vi "BASE-Julian Code.vi"() -> (0 "Long Date":string, 1 "Short Date":string, 2 "Shift":string, 3 "Julian Code":string, 4 "Long time with :":string, 5 "Long date with /":string)   [LabVIEW 2017]
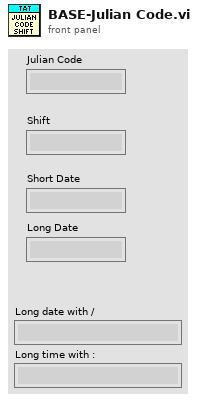
[diagram p1: front panel]
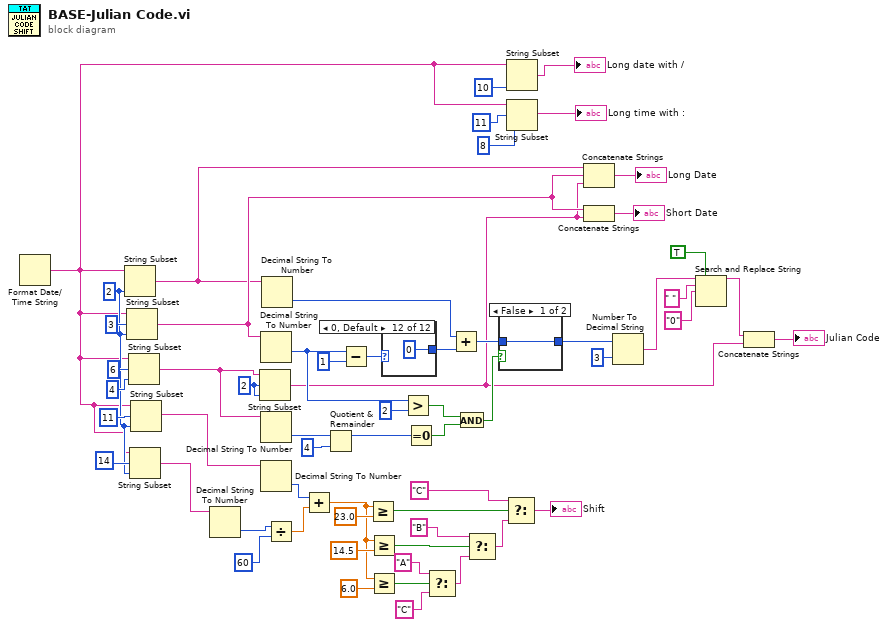
[diagram p0: block diagram]
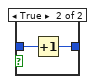
[diagram p2: hidden frame]
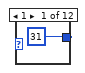
[diagram p3: hidden frame]
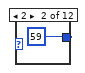
[diagram p4: hidden frame]
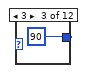
[diagram p5: hidden frame]
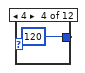
[diagram p6: hidden frame]
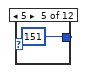
[diagram p7: hidden frame]
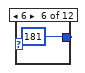
[diagram p8: hidden frame]
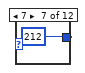
[diagram p9: hidden frame]
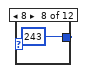
[diagram p10: hidden frame]
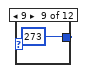
[diagram p11: hidden frame]
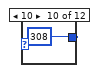
[diagram p12: hidden frame]
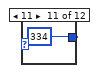
[diagram p13: hidden frame]
diagram:
  w32 = 2 ("length (rest)")
  w60 = 2 ("offset (0)")
  n1 = Format Date/Time String() -> (date/time string=w3:string)  [unwired: 3 in]
  n2 = String Subset(string=w3, length (rest)=w32) -> (substring=w7:string)  [unwired: 1 in]
  n3 = String Subset(string=w3, offset (0)=3, length (rest)=w32) -> (substring=w9:string)
  n4 = String Subset(string=w3, offset (0)=6, length (rest)=4 ("length (rest)")) -> (substring=w47:string)
  n5 = String Subset(string=w3, offset (0)=14, length (rest)=w32) -> (substring=w31:string)
  n6 = String Subset(string=w3, offset (0)=11, length (rest)=w32) -> (substring=w25:string)
  n7 = Decimal String To Number(string=w31) -> (number=w30:i32)  [unwired: 2 in, 1 out]
  n8 = String Subset(string=w47, offset (0)=w60, length (rest)=w60) -> (substring=w8:string)
  n9 = Decimal String To Number(string=w9) -> (number=w18:i32)  [unwired: 2 in, 1 out]
  n10 = Decimal String To Number(string=w47) -> (number=w59:i32)  [unwired: 2 in, 1 out]
  n11 = Decimal String To Number(string=w25) -> (number=w28:i32)  [unwired: 2 in, 1 out]
  n12 = Decimal String To Number(string=w7) -> (number=w54:i32)  [unwired: 2 in, 1 out]
  n13 = Divide(x=w30, y=60) -> (x/y=w27:dbl)
  n14 = Add(x=w28, y=w27) -> (x+y=w26:dbl)
  n15 = Quotient & Remainder(x=w59, y=4) -> (x-y*floor(x/y)=w57:i32)  [unwired: 1 out]
  n16 = Subtract(x=w18, y=1) -> (x-y=w55:i32)
  n17 = Greater Or Equal?(x=w26, y=23.0) -> (x >= y?=w43:bool)
  n18 = Greater Or Equal?(x=w26, y=14.5) -> (x >= y?=w35:bool)
  n19 = Greater Or Equal?(x=w26, y=6.0) -> (x >= y?=w38:bool)
  n20 = case shown="0, Default" w55 {
    tunnel: [31 ("y") 59 ("y") 90 ("y") 120 ("y") 151 ("y") 181 ("y") 212 ("y") 243 ("y") 273 ("y") 308 ("y") 334 ("y") 0 ("y")] -> w53
    frame 1 {
    }
    frame 2 {
    }
    frame 3 {
    }
    frame 4 {
    }
    frame 5 {
    }
    frame 6 {
    }
    frame 7 {
    }
    frame 8 {
    }
    frame 9 {
    }
    frame 10 {
    }
    frame 11 {
    }
    frame 0, Default {
    }
  }
  n21 = Greater?(x=w18, y=2) -> (0:w16:bool)
  n22 = Equal To 0?(x=w57) -> (x = 0?=w15:bool)
  n23 = Select(t="A", s=w38, f="C") -> (s? t:f=w40:string)
  n24 = Add(x=w54, y=w53) -> (x+y=w20:i32)
  n25 = And(x=w16, y=w15) -> (x .and. y?=w14:bool)
  n26 = Select(t="B", s=w35, f=w40) -> (s? t:f=w41:string)
  n27 = case shown="False" w14 {
    tunnel: w20 -> [w73 w75]
    tunnel: [w73 w74] -> w19
    frame False {
    }
    frame True {
      n28 = Increment(x=w75) -> (x+1=w74:i32)
    }
  }
  n29 = Select(t="C", s=w43, f=w41) -> (s? t:f=→"Shift":string)
  n30 = String Subset(string=w3, length (rest)=10 ("length (rest)")) -> (substring=→"Long date with /":string)  [unwired: 1 in]
  n31 = String Subset(string=w3, offset (0)=11 ("length (rest)"), length (rest)=8 ("length (rest)")) -> (substring=→"Long time with :":string)
  n32 = Concatenate Strings(w7, w9, w8) -> (→"Long Date":string)
  n33 = Concatenate Strings(w9, w8) -> (→"Short Date":string)
  n34 = Number To Decimal String(number=w19, width (-)=i16 3) -> (decimal integer string=w23:string)
  n35 = Search and Replace String(replace all?=TRUE ("replace all? (F)"), input string=w23, search string=" ", replace string="0" ("replace string (\"\")")) -> (result string=w13:string)  [unwired: 4 in, 3 out]
  n36 = Concatenate Strings(w13, w8) -> (→"Julian Code":string)
